vi "Module Measure Filter.vi"(8 "error in":errorcluster, 9 "MeasType":T2=enum."Dynamic", 10 "Rate Class":T1, 11 "Module Name":string) -> (0 "error out":errorcluster, 3 "Mod Pass":bool)   [LabVIEW 2018]
uses:
  Custom Ctrls/ge_MeasType.ctl
  Common/Controls/TE_Designator.ctl
  Common/Controls/Timing Engine Support.ctl
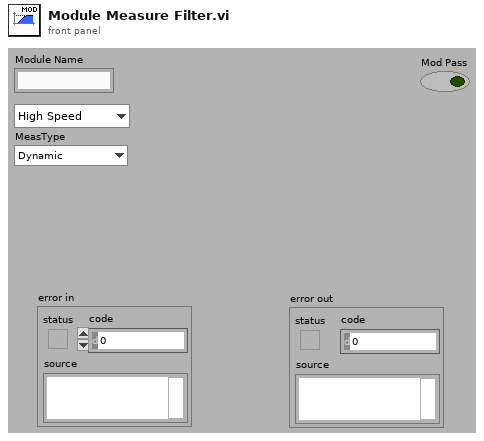
[diagram p1: front panel]
types:
  T1 = typedef "TE_Designator.ctl" = enum16{"High Speed", "Low Speed"}
  T2 = typedef "ge_MeasType.ctl" = enum16{"Voltage", "Frequency", "Tachometer", "Dynamic", "Thermocouple", "RTD", "Strain", "Current", "Resistance"}
  T3 = typedef "Timing Engine Support.ctl" = enum16{"HS Mod", "LS Mod", "Either"}
  T4 = typedef "DAQMan Definitions.ctl" = cluster{"Timing Engine Defs":variant, "Table Definitions":variant, "Ring Definitions":variant}
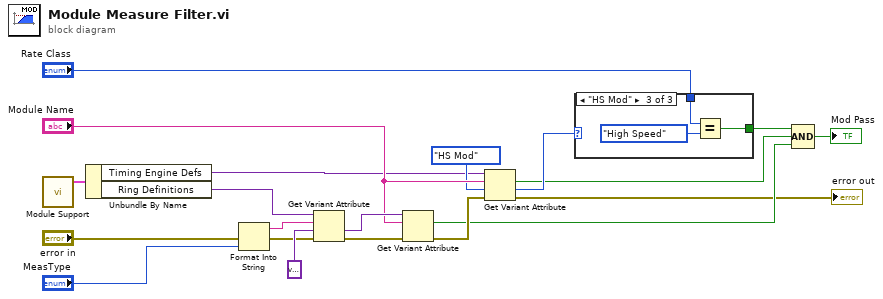
[diagram p0: block diagram]
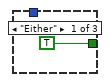
[diagram p2: hidden frame]
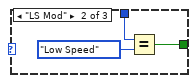
[diagram p3: hidden frame]
diagram:
  n1 = call "Module Support.vi"() -> ("ge_DAQManDefinitions"=w1:T4)  [unwired: 9 in]
  n2 = Unbundle By Name(w1) -> ("Timing Engine Defs"=w4:variant, "Ring Definitions"=w5:variant)
  n3 = Format Into String(error in="error in", "MeasType") -> (resulting string=w19:string, error out=w17:errorcluster)  [unwired: 2 in]
  n4 = Get Variant Attribute(Variant=w5, name=w19, default value (empty Variant)=variant ("default value (empty variant)"), error in=w17) -> (value=w15:variant, error out=w16:errorcluster)  [unwired: 2 out]
  n5 = Get Variant Attribute(Variant=w15, name="Module Name", error in=w16) -> (found=w9:bool, error out=w14:errorcluster)  [unwired: 1 in, 2 out]
  n6 = Get Variant Attribute(Variant=w4, name="Module Name", default value (empty Variant)=Timing_Engine_Support."HS Mod" ("ValidRates"), error in=w14) -> (found=w6:bool, value=w10:T3, error out=→"error out":errorcluster)  [unwired: 1 out]
  n7 = case shown="\"HS Mod\"" w10 {
    tunnel: "Rate Class" -> [_ w24 w27]
    tunnel: [TRUE w22 w25] -> w7
    frame "Either" {
    }
    frame "LS Mod" {
      n8 = Equal?(x=w24, y=TE_Designator."Low Speed") -> (x = y?=w22:bool)
    }
    frame "HS Mod" {
      n9 = Equal?(x=w27, y=TE_Designator."High Speed") -> (x = y?=w25:bool)
    }
  }
  n10 = Compound Arithmetic op=AND(w7, w6, w9) -> (→"Mod Pass":bool)
